vi "Set Default Values.vi"(8 "error in (no error)":errorcluster, 10 "App Config":path, 11 "Step in":refnum<class "Step.lvclass">) -> (0 "error out":errorcluster, 3 "Step out":refnum<class "Step.lvclass">)   [LabVIEW 2020, in "MacroAssert.lvlib" / "Step.lvclass"]
uses:
  Step.lvclass
  <vilib>/Utility/config.llb/NI_LVConfig.lvlib
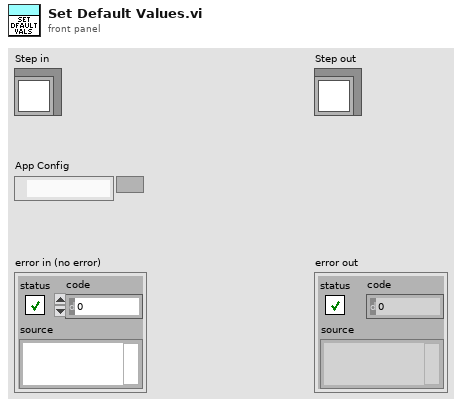
[diagram p1: front panel]
types:
  T1 = typedef "MacroAssert.lvlib/Step Type V3.ctl" = enum16{"Mouse Action", "Keyboard Action", "Window Action", "Timing Action", "Boolean Assertion", "Numeric Assertion", "String Assertion", "Image Assertion"}
  T2 = typedef "NI_LVConfig.lvlib/Config Data RefNum.ctl" = refnum<k1>
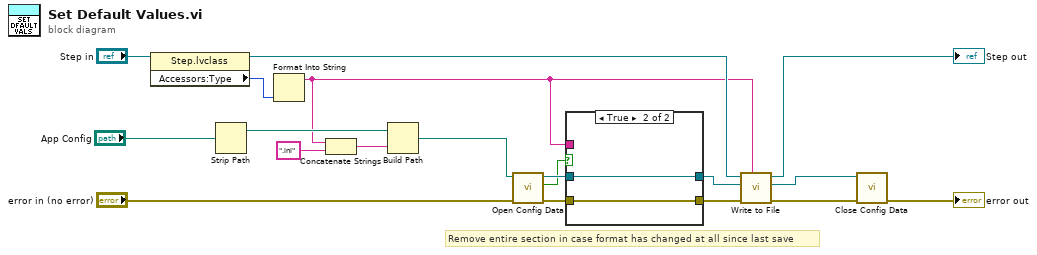
[diagram p0: block diagram]
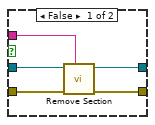
[diagram p2: hidden frame]
diagram:
  # "Remove entire section in case format has changed at all since last save"
  n1 = property class="Step.lvclass"(reference="Step in") -> (reference out=w16:refnum<class "Step.lvclass">, "Accessors:Type"=w13:T1)  [unwired: 1 in, 1 out]
  n2 = Strip Path(path="App Config") -> (stripped path=w14:path)  [unwired: 1 out]
  n3 = Format Into String(w13) -> (resulting string=w2:string)  [unwired: 3 in, 1 out]
  n4 = Concatenate Strings(w2, ".ini" ("format string")) -> (w10:string)
  n5 = Build Path(base path=w14, name or relative path=w10) -> (appended path=w11:path)
  n6 = call <vilib>:"Open Config Data.vi"("error in (no error)"="error in (no error)", "configuration file path"=w11) -> ("error out"=w6:errorcluster, "file created?"=w1:bool, "refnum"=w4:T2)  [unwired: 7 in]
  n7 = case shown="True" w1 {
    tunnel: w6 -> [w24 w25]
    tunnel: [w23 w25] -> w5
    tunnel: w4 -> [w22 w26]
    tunnel: [w21 w26] -> w3
    tunnel: w2 -> [w20 _]
    frame False {
      n8 = call <vilib>:"Remove Section.vi"("section"=w20, "error in (no error)"=w24, "refnum"=w22) -> ("error out"=w23:errorcluster, "refnum out"=w21:T2)  [unwired: 6 in, 1 out]
    }
    frame True {
    }
  }
  n9 = call-dynamic "Write to File.vi"("Section Name"=w2, "error in (no error)"=w5, "INI Ref"=w3, "Step in"=w16) -> ("error out"=w8:errorcluster, "INI Ref out"=w7:T2, "Step out"=→"Step out":refnum<class "Step.lvclass">)  [unwired: 5 in]
  n10 = call <vilib>:"Close Config Data.vi"("error in (no error)"=w8, "refnum"=w7) -> ("error out"=→"error out":errorcluster)  [unwired: 8 in, 1 out]
